vi "Elevator - Send Command.vi"(8 "error in (no error)":errorcluster, 9 "Variant":variant, 10 "Elevator Commands":T1, 11 "View Model":T2) -> (0 "error out":errorcluster, 3 "View Model":T2)   [LabVIEW 2017]
doc: "Generates user event and send command with parameters to elevator controlle."
uses:
  View Model/Controls/View Model.ctl
  Configuration/Controls/Config Model.ctl
  Configuration/Controls/Config Data.ctl
  Error Handler/Controls/Error Model.ctl
  Error Handler/Controls/Error Data.ctl
  Error Handler/Controls/Error Type.ctl
  View Model/Controls/Shared Model.ctl
  Controls/Elevator Model.ctl
  Controls/Elevator Location.ctl
  Controls/Elevator CMD Data.ctl
  Controls/Elevator Commands.ctl
  Controls/Elevator Overhead.ctl
  Controls/Elevator States.ctl
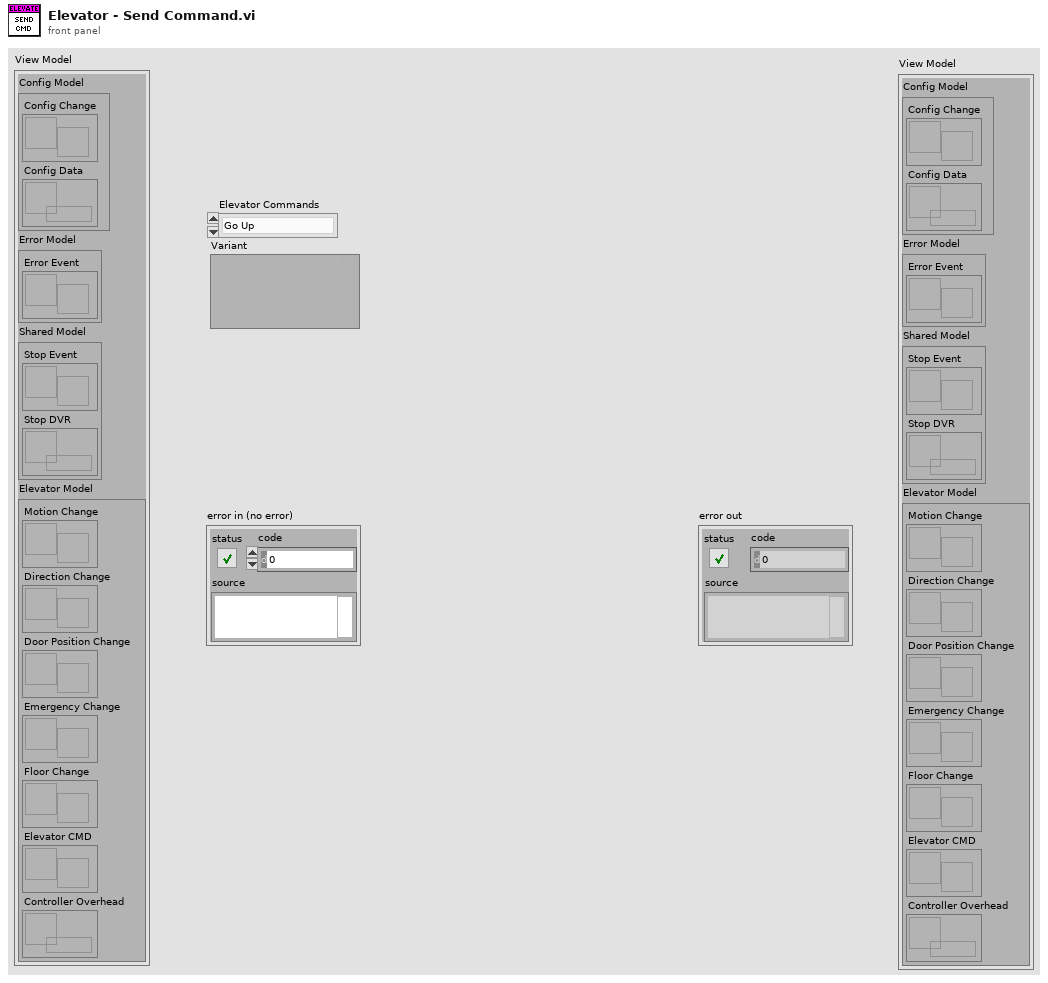
[diagram p1: front panel]
types:
  T1 = typedef "Elevator Commands.ctl" = enum16{"Go Up", "Go Down", "Go to Floor", "Emergency", "Open Doors", "Close Doors"}
  T2 = typedef "View Model.ctl" = cluster{"Config Model":T3, "Error Model":T4, "Shared Model":T5, "Elevator Model":T6}
  T3 = typedef "Config Model.ctl" = cluster{"Config Change":refnum<user-event>, "Config Data":refnum<data-value>}
  T4 = typedef "Error Model.ctl" = cluster{"Error Event":refnum<user-event>}
  T5 = typedef "Shared Model.ctl" = cluster{"Stop Event":refnum<user-event>, "Stop DVR":refnum<data-value>}
  T6 = typedef "Elevator Model.ctl" = cluster{"Motion Change":refnum<user-event>, "Direction Change":refnum<user-event>, "Door Position Change":refnum<user-event>, "Emergency Change":refnum<user-event>, "Floor Change":refnum<user-event>, "Elevator CMD":refnum<user-event>, "Controller Overhead":refnum<data-value>}
  T7 = typedef "Elevator CMD Data.ctl" = cluster{"Elevator Commands":T1, "Variant":variant}
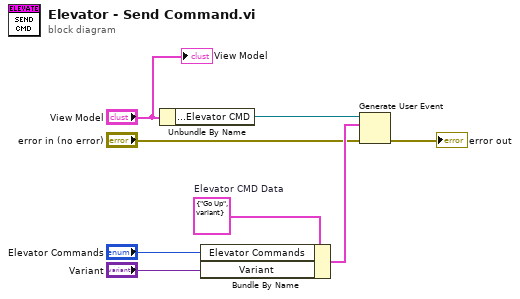
[diagram p0: block diagram]
diagram:
  w6 = T7 {"Elevator Commands"=enum."Go Up", "Variant"=variant}  # Elevator CMD Data
  n1 = Unbundle By Name("View Model") -> ("Elevator Model.Elevator CMD"=w8:refnum<user-event>)
  n2 = Bundle By Name(cluster=w6, "Elevator Commands"="Elevator Commands", "Variant"="Variant") -> (w3:T7)
  n3 = Generate User Event(user event=w8, event data cluster=w3, error in="error in (no error)") -> (error out=→"error out":errorcluster)  [unwired: 1 in, 1 out]
  "View Model" <- "View Model"
